vi "Read Config_INI_String.vi"(0 "refnum":T1, 1 "section":string, 9 "Keys":string[](array[string]), 11 "error in (no error)":errorcluster) -> (4 "refnum out":T1, 10 "Outputs":string[](array[string]), 15 "error out":errorcluster)   [LabVIEW 2017]
uses:
  <vilib>/Utility/config.llb/Config Data RefNum.ctl
  <vilib>/Utility/config.llb/Read Key (String).vi
  <vilib>/Utility/config.llb/NI_LVConfig.lvlib
panel:
  out "Outputs 2":string[](array[string])
  in  "key":string
  out "refnum out 2":T1 caption="配置数据"
  in  "refnum 2":T1 caption="配置数据"
  in  "section 2":string
  in  "error in (no error) 2":errorcluster
  out "error out 2":errorcluster
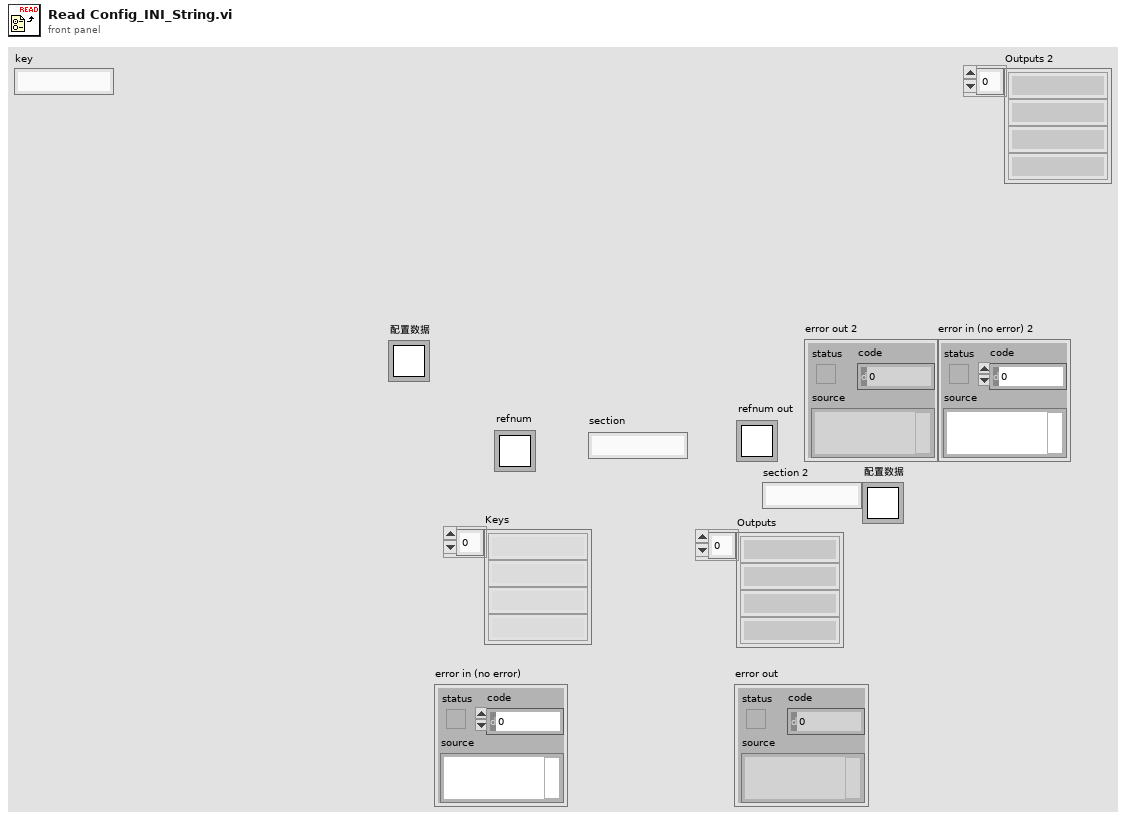
[diagram p1: front panel]
types:
  T1 = typedef "NI_LVConfig.lvlib/Config Data RefNum.ctl" = refnum<k1>
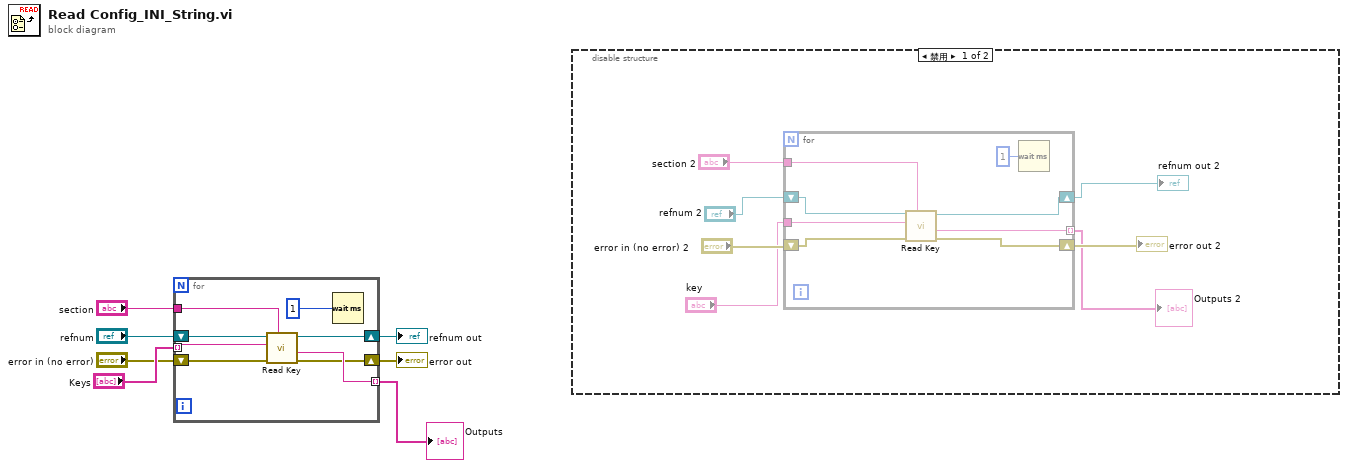
[diagram p0: block diagram]
diagram:
  n1 = for {
    tunnel: "section" -> [w13]
    shift-right: [w14] -> w6
    shift-left: "refnum" -> [w15]
    tunnel: "Keys" -> [w12] mode=indexing
    tunnel: [w11] -> w1 mode=indexing
    shift-right: [w9] -> w3
    shift-left: "error in (no error)" -> [w8]
    n2 = call-poly <vilib>:"Read Key.vi"("section"=w13, "error in (no error)"=w8, "key"=w12, "refnum"=w15) -> ("error out"=w9:errorcluster, "value"=w11:string, "refnum out"=w14:T1)  [unwired: 4 in, 1 out]
    n3 = Wait (ms)(milliseconds to wait=u32 1) -> ()  [unwired: 1 out]
  }
  "refnum out" <- w6
  "error out" <- w3
  "Outputs" <- w1
  n4 = disable-structure shown="禁用" {
    frame Disabled {
      n5 = for {
        shift-right: [w28] -> w21
        shift-left: "error in (no error) 2" -> [w29]
        tunnel: "section 2" -> [w27]
        shift-right: [w25] -> w18
        shift-left: "refnum 2" -> [w26]
        tunnel: "key" -> [w24]
        tunnel: [w23] -> w16 mode=indexing
        n6 = call-poly <vilib>:"Read Key.vi"("section"=w27, "error in (no error)"=w29, "key"=w24, "refnum"=w26) -> ("error out"=w28:errorcluster, "value"=w23:string, "refnum out"=w25:T1)  [unwired: 4 in, 1 out]
        n7 = Wait (ms)(milliseconds to wait=u32 1 ("等待时间（毫秒）")) -> ()  [unwired: 1 out]
      }
      "error out 2" <- w21
      "refnum out 2" <- w18
      "Outputs 2" <- w16
    }
    frame Enabled {
    }
  }
